vi "InitLogging.vi"(8 "error in (no error)":errorcluster, 11 "AppDataPath":path) -> (0 "error out":errorcluster, 2 "clLogging":T1={"eLogLvl"=enum."Normal", "Log File Path"=path "", "btnLogFile"=FALSE}, 3 "AppDataPath":path)   [LabVIEW 2017, in "Framework.lvlib" / "Config.lvclass"]
uses:
  Config.lvclass
  Typedefs/Logging.ctl
  Typedefs/eLogLvl.ctl
  <vilib>/Utility/config.llb/NI_LVConfig.lvlib
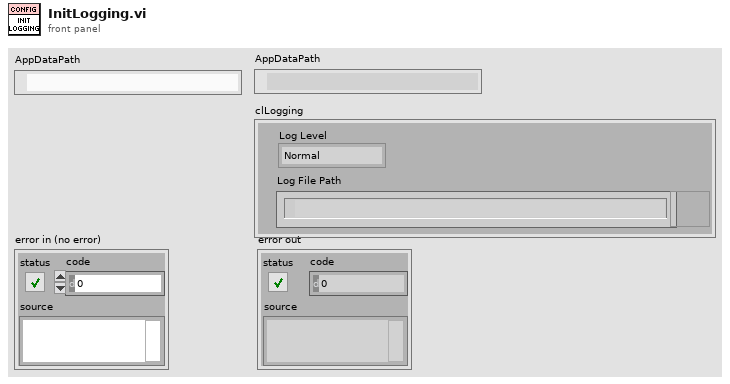
[diagram p1: front panel]
types:
  T1 = typedef "Framework.lvlib/Config.lvclass/Logging.ctl" = cluster{"eLogLvl":T2, "Log File Path":path, "btnLogFile":bool}
  T2 = typedef "Framework.lvlib/Config.lvclass/eLogLvl.ctl" = enum16{"Normal", "Verbose", "None"}
  T3 = typedef "NI_LVConfig.lvlib/Config Data RefNum.ctl" = refnum<k1>
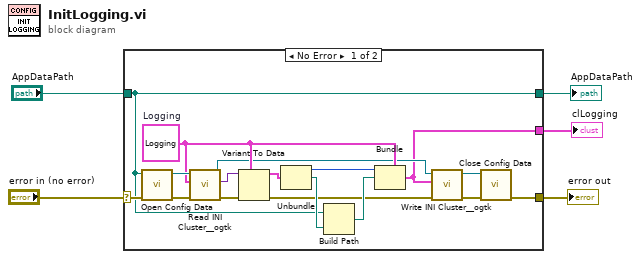
[diagram p0: block diagram]
diagram:
  n1 = case shown="No Error" "error in (no error)" {
    selector: "error in (no error)" -> [w8 w24]
    tunnel: [w9 _] -> w5
    tunnel: "AppDataPath" -> [w6 w23]
    tunnel: [w7 w24] -> w2
    tunnel: [w6 w23] -> w1
    frame No Error {
      w17 = T1 {"eLogLvl"=enum."Verbose", "Log File Path"=path "C:/Users/gra1/AppData/Local/Framework/Framework.log", "btnLogFile"=FALSE}  # Logging
      n2 = call <vilib>:"Open Config Data.vi"("error in (no error)"=w8, "configuration file path"=w6) -> ("error out"=w22:errorcluster, "refnum"=w21:T3)  [unwired: 7 in, 1 out]
      n3 = call <userlib>:"Read INI Cluster__ogtk.vi"("error in (no error)"=w22, "INI Fomatted Cluster Type"=w17, "refnum"=w21) -> ("error out"=w20:errorcluster, "INI Fomatted Cluster"=w19:variant, "dup refnum"=w11:T3)  [unwired: 4 in, 2 out]
      n4 = Variant To Data(error in=w20, type=w17, Variant=w19) -> (data=w18:T1, error out=w13:errorcluster)
      n5 = Unbundle(w18) -> ("eLogLvl"=w16:T2, "Log File Path"=w15:path)  [unwired: 1 out]
      n6 = Build Path(base path=w6, name or relative path=w15) -> (appended path=w14:path)
      n7 = Bundle(cluster=w17, "eLogLvl"=w16, "Log File Path"=w14) -> (w9:T1)  [unwired: 1 in]
      n8 = call <userlib>:"Write INI Cluster__ogtk.vi"("error in (no error)"=w13, "INI Fomatted Cluster"=w9, "refnum"=w11) -> ("error out"=w12:errorcluster, "dup refnum"=w10:T3)  [unwired: 7 in]
      n9 = call <vilib>:"Close Config Data.vi"("error in (no error)"=w12, "refnum"=w10) -> ("error out"=w7:errorcluster)  [unwired: 8 in, 1 out]
    }
    frame Error {
    }
  }
  "error out" <- w2
  "AppDataPath" <- w1
  "clLogging" <- w5
